vi "Pre Launch Init.vi"(11 "Connection Listener in":refnum<class "Connection Listener.lvclass">) -> (0 "error out":errorcluster, 3 "Connection Listener out":refnum<class "Connection Listener.lvclass">)   [LabVIEW 2017, in "Connection Listener.lvlib" / "Connection Listener.lvclass"]
doc: "(<B>Filename</B>: Actor Framework.lvlib:Actor.lvclass:Pre Launch Init.vi)\n\nDefines behavior that occurs after the Launch Nested Actor method is invoked but before the actor's Actor Core method begins running.\n\nBy default, this method does nothing. A descendant class may override it to define behavior."
uses:
  Connection Listener.lvclass
  Connection Listener.lvclass/Connection Listener.ctl
  <vilib>/MediaMongrels Ltd/WebSockets/Sockets/VISA TCP Listener/VISA TCP Listener.lvclass
  Framework/Actor wHelper/Actor wHelper.lvclass
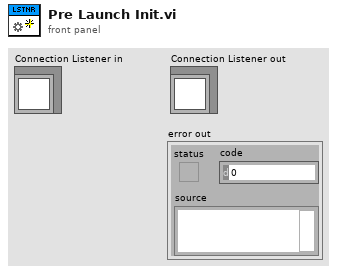
[diagram p1: front panel]
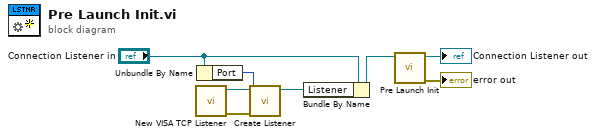
[diagram p0: block diagram]
diagram:
  n1 = call <vilib>:"New VISA TCP Listener.vi"() -> ("error out"=w3:errorcluster, "VISA TCP Listener out"=w5:refnum<class "VISA TCP Listener.lvclass">)  [unwired: 10 in]
  n2 = Unbundle By Name("Connection Listener in") -> ("Port"=w1:u16)
  n3 = call-dynamic "Create Listener.vi"("error in (no error)"=w3, "Port"=w1, "VISA TCP Listener in"=w5) -> ("VISA TCP Listener out"=w4:refnum<class "VISA TCP Listener.lvclass">)  [unwired: 7 in, 1 out]
  n4 = Bundle By Name(cluster="Connection Listener in", "Listener"=w4) -> (w6:refnum<class "Connection Listener.lvclass">)
  n5 = call-parent "Pre Launch Init.vi"("Actor wHelper in"=w6) -> ("error out"=→"error out":errorcluster, "Actor wHelper out"=→"Connection Listener out":refnum<class "Connection Listener.lvclass">)  [unwired: 9 in]
